vi "funcArgChk.vi"(8 "error in":errorcluster, 9 "Row number":u32, 10 "Tbl Refnum in":refnum<vi>, 11 "Tree Refnum in":refnum<vi>) -> (0 "error out":errorcluster, 1 "Check result":string="√", 2 "Tbl Refnum out":refnum<vi>, 3 "Tree Refnum out":refnum<vi>)   [LabVIEW 2010]
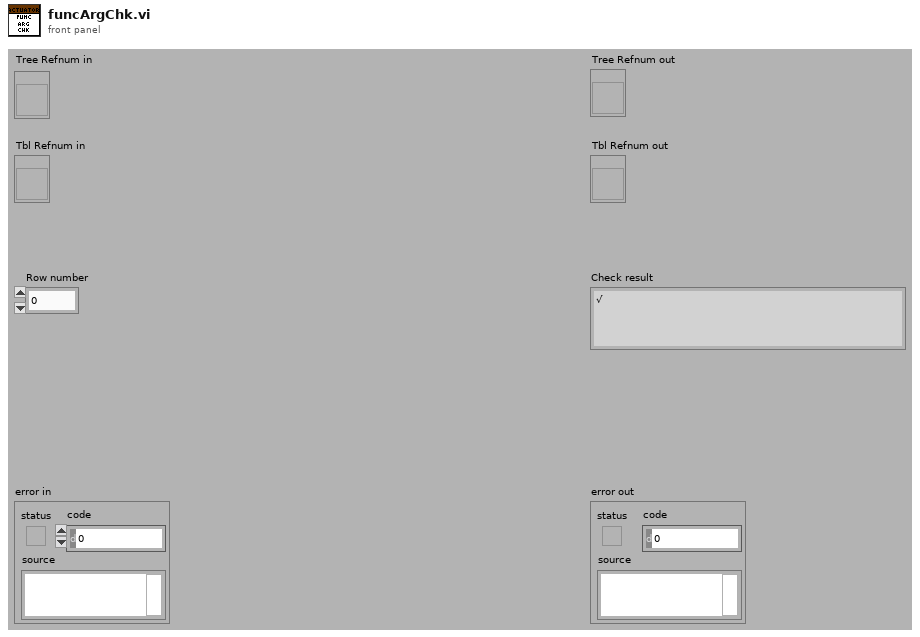
[diagram p1: front panel]
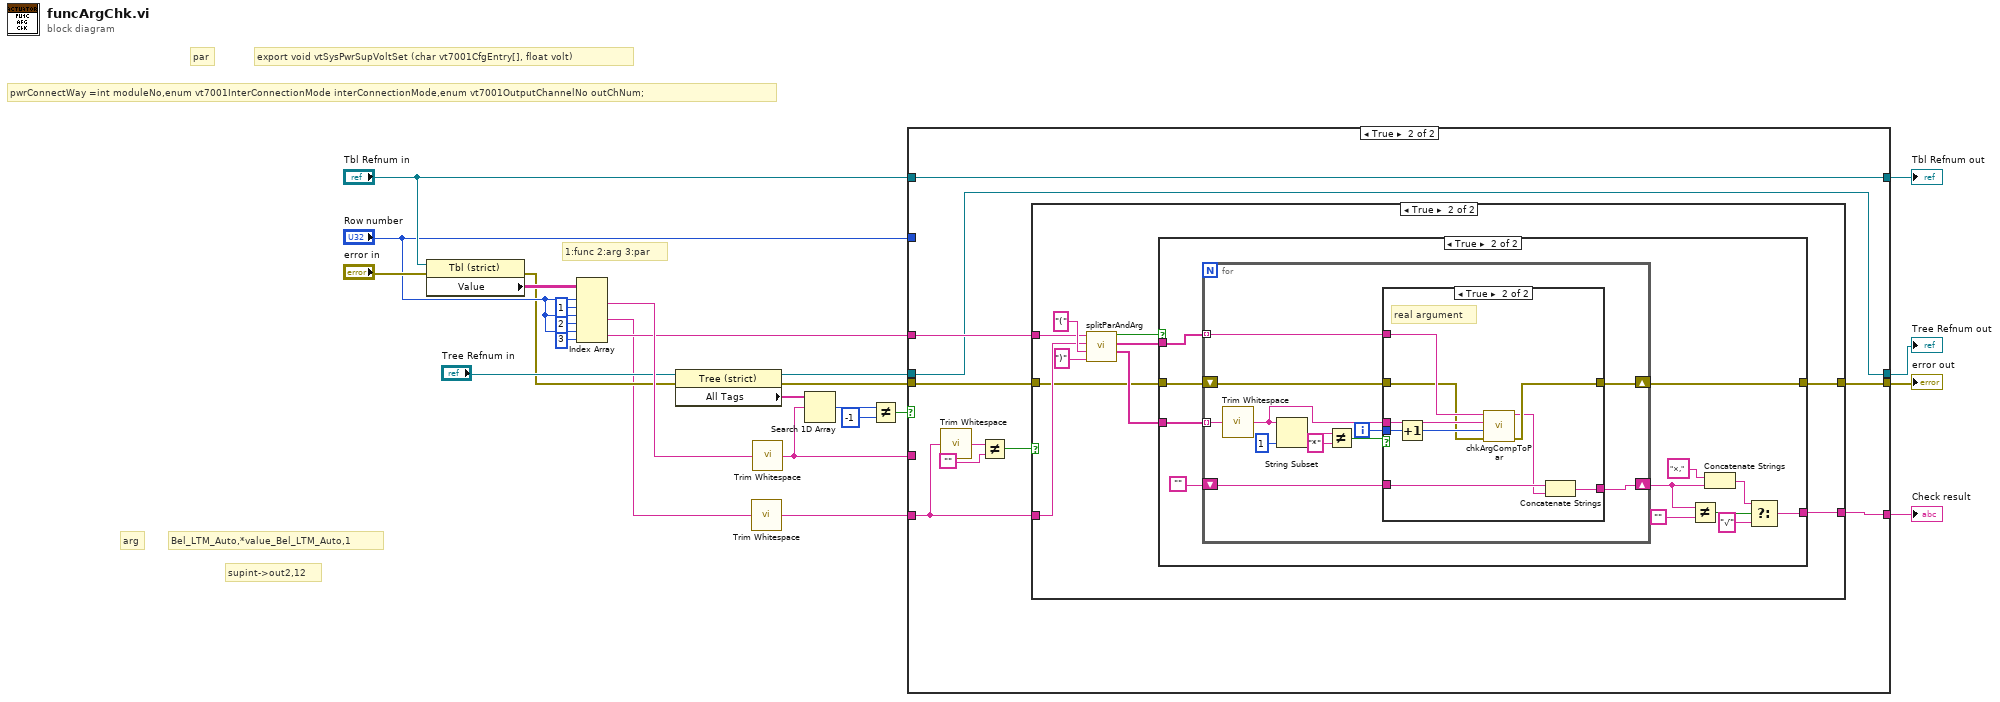
[diagram p0: block diagram]
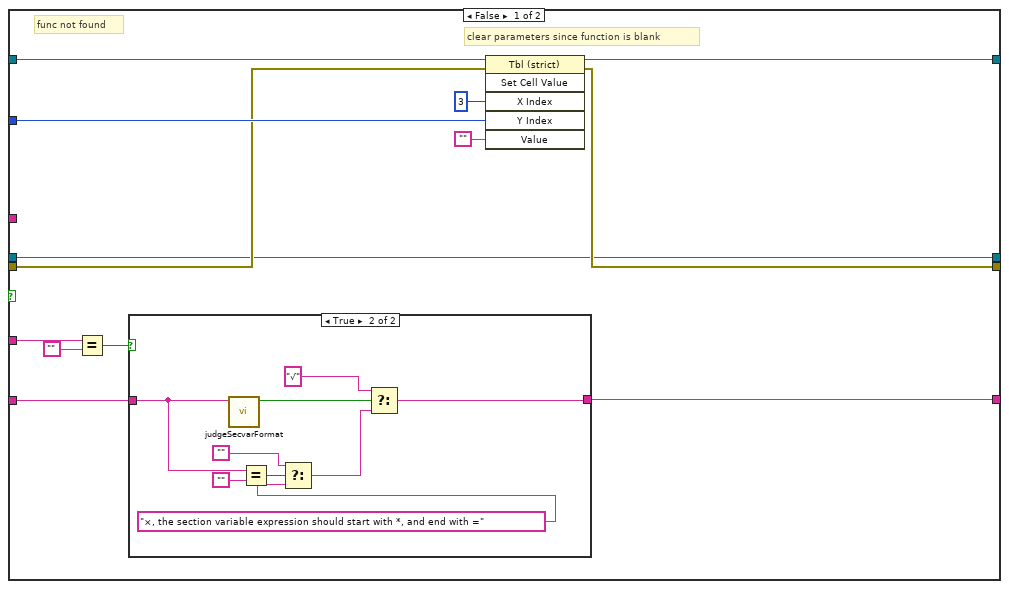
[diagram p2: hidden frame]
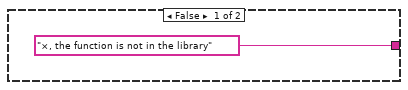
[diagram p3: hidden frame]
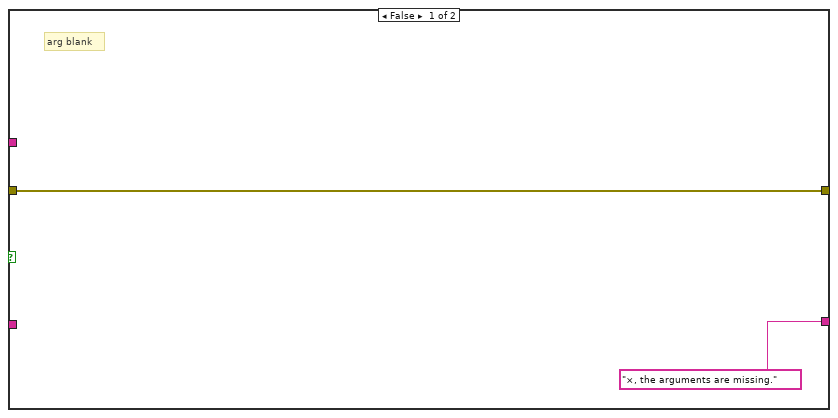
[diagram p4: hidden frame]
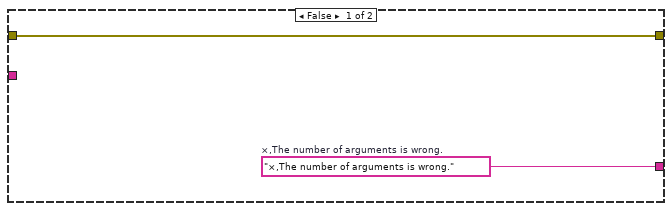
[diagram p5: hidden frame]
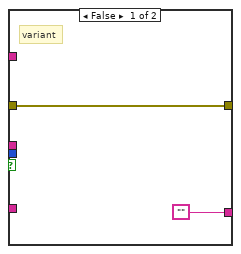
[diagram p6: hidden frame]
diagram:
  # "pwrConnectWay =int moduleNo,enum vt7001InterConnectionMode interConnectionMode,enum vt7001OutputChannelNo outChNum;"
  # "arg"
  # "par"
  # "1:func 2:arg 3:par"
  # "Bel_LTM_Auto,*value_Bel_LTM_Auto,1"
  # "supint->out2,12"
  # "export void vtSysPwrSupVoltSet (char vt7001CfgEntry[], float volt)"
  n1 = property class="Tbl (strict)"(reference="Tbl Refnum in", error in="error in") -> (error out=w4:errorcluster, "Value"=w13:string[][])  [unwired: 1 out]
  n2 = Index Array(array=w13, index (row) #1="Row number", index (col) #1=1 ("disabled index (col)"), index (row) #2="Row number", index (col) #2=2 ("index (col)"), index (row) #3="Row number", index (col) #3=3 ("disabled index (col)")) -> (element #1=w7:string, element #2=w1:string, element #3=w6:string)
  n3 = property on="Property Node" class="Tree (strict)"(reference="Tree Refnum in", error in=w4) -> (reference out=w16:refnum<vi>, error out=w17:errorcluster, "All Tags"=w20:string[])
  n4 = call <vilib>:"Trim Whitespace.vi"("string"=w1) -> ("trimmed string"=w2:string)  [unwired: 1 in]
  n5 = call <vilib>:"Trim Whitespace.vi"("string"=w7) -> ("trimmed string"=w3:string)  [unwired: 1 in]
  n6 = Search 1D Array(1D array=w20, element=w3) -> (index of element=w19:i32)  [unwired: 1 in]
  n7 = Not Equal?(x=w19, y=-1) -> (x != y?=w24:bool)
  n8 = case shown="True" w24 {
    tunnel: w6 -> [_ w57]
    tunnel: w2 -> [w27 w50]
    tunnel: w17 -> [w31 w56]
    tunnel: [w26 w55] -> w23
    tunnel: [w34 w54] -> w22
    tunnel: "Tbl Refnum in" -> [w32 w48]
    tunnel: "Row number" -> [w33 _]
    tunnel: [w35 w48] -> w21
    tunnel: w16 -> [w25 w49]
    tunnel: [w25 w49] -> w15
    tunnel: w3 -> [w30 _]
    frame False {
      # "clear parameters since function is blank"
      # "func not found"
      n9 = Equal?(x=w30, y="") -> (x = y?=w28:bool)
      n10 = case shown="True" w28 {
        tunnel: w27 -> [_ w40]
        tunnel: ["×, the function is not in the library" w46] -> w26
        frame False {
        }
        frame True {
          n11 = call "judgeSecvarFormat.vi"("section variable"=w40) -> ("correct format?"=w41:bool)  [unwired: 10 in]
          n12 = Equal?(x=w40, y="") -> (x = y?=w45:bool)
          n13 = Select(t="", s=w45, f="×, the section variable expression should start with *, and end with =" ("Value")) -> (s? t:f=w39:string)
          n14 = Select(t="√", s=w41, f=w39) -> (s? t:f=w46:string)
        }
      }
      n15 = invoke class="Tbl (strict)" method="Set Cell Value"(reference=w32, error in=w31, "X Index"=u32 3, "Y Index"=w33, "Value"="") -> (reference out=w35:refnum<vi>, error out=w34:errorcluster)  [unwired: 1 in, 4 out]
    }
    frame True {
      n16 = call <vilib>:"Trim Whitespace.vi"("string"=w50) -> ("trimmed string"=w53:string)  [unwired: 1 in]
      n17 = Not Equal?(x=w53, y="") -> (x != y?=w51:bool)
      n18 = case shown="True" w51 {
        tunnel: w57 -> [_ w65]
        tunnel: w50 -> [_ w64]
        tunnel: w56 -> [w59 w60]
        tunnel: ["×, the arguments are missing." w69] -> w55
        tunnel: [w59 w68] -> w54
        frame False {
          # "arg blank"
        }
        frame True {
          n19 = call "splitParAndArg.vi"("paraEndMark"=")" ("regular expression"), "paraStartMark"="(" ("regular expression"), "allArguments"=w64, "allParameters"=w65) -> ("argArray"=w62:string[], "paraArray"=w63:string[], "sameNum?"=w61:bool)  [unwired: 5 in]
          n20 = case shown="True" w61 {
            tunnel: w63 -> [_ w83]
            tunnel: w62 -> [_ w82]
            tunnel: [w71 w77] -> w69
            tunnel: w60 -> [w70 w76]
            tunnel: [w70 w75] -> w68
            frame False {
              w71 = "×,The number of arguments is wrong."  # ×,The number of arguments is wrong.
            }
            frame True {
              n21 = for {
                tunnel: w83 -> [w95] mode=indexing
                tunnel: w82 -> [w85] mode=indexing
                shift-right: [w93] -> w73
                shift-left: "" -> [w94]
                shift-right: [w91] -> w75
                shift-left: w76 -> [w92]
                i -> [w86]
                n22 = call <vilib>:"Trim Whitespace.vi"("string"=w85) -> ("trimmed string"=w84:string)  [unwired: 1 in]
                n23 = String Subset(string=w84, length (rest)=1 ("length (rest)")) -> (substring=w89:string)  [unwired: 1 in]
                n24 = Not Equal?(x=w89, y="*") -> (x != y?=w87:bool)
                n25 = case shown="True" w87 {
                  tunnel: w95 -> [_ w103]
                  tunnel: w94 -> [_ w106]
                  tunnel: ["" w105] -> w93
                  tunnel: w92 -> [w96 w100]
                  tunnel: [w96 w99] -> w91
                  tunnel: w86 -> [_ w102]
                  tunnel: w84 -> [_ w104]
                  frame False {
                    # "variant"
                  }
                  frame True {
                    # "real argument"
                    n26 = Increment(x=w102) -> (x+1=w101:i32)
                    n27 = call "chkArgCompToPar.vi"("error in"=w100, "argSN"=w101, "arg"=w104, "par"=w103) -> ("error out"=w99:errorcluster, "judgement"=w98:string)  [unwired: 6 in]
                    n28 = Concatenate Strings(w106, w98) -> (w105:string)
                  }
                }
              }
              n29 = Not Equal?(x=w73, y="") -> (x != y?=w79:bool)
              n30 = Concatenate Strings("×,", w73) -> (w72:string)
              n31 = Select(t=w72, s=w79, f="√") -> (s? t:f=w77:string)
            }
          }
        }
      }
    }
  }
  "Check result" <- w23
  "error out" <- w22
  "Tbl Refnum out" <- w21
  "Tree Refnum out" <- w15
